vi "All stations screw ID config.vi"(10 "station idx":i32, 11 "configuration file path":path) -> (0 "error out":errorcluster caption="错误输出", 2 "station idx":i32, 3 "configuration file path":path, 5 "Screw config":T1)   [LabVIEW 2018]
uses:
  Crl defs/one state screw config.ctl
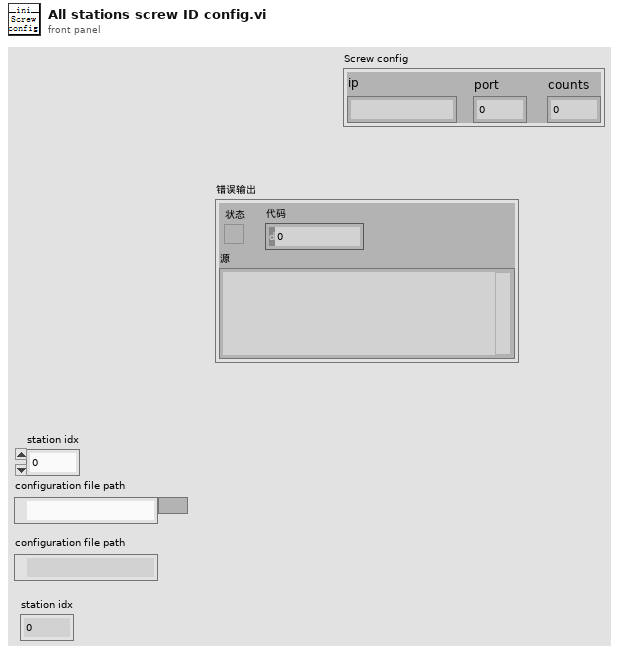
[diagram p1: front panel]
types:
  T1 = typedef "one state screw config.ctl" = cluster{"ip":string, "port":u16, "counts":u16}
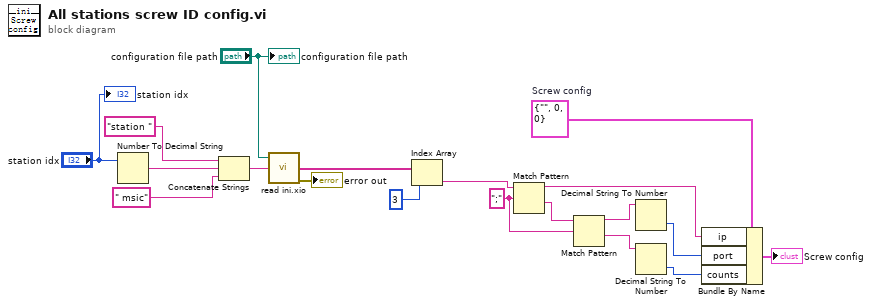
[diagram p0: block diagram]
diagram:
  w7 = T1 {"ip"="", "port"=0, "counts"=0}  # Screw config
  w9 = ";" ("正则表达式")
  n1 = Number To Decimal String(number="station idx") -> (decimal integer string=w17:string)  [unwired: 1 in]
  n2 = Concatenate Strings("station ", w17, " msic" ("string")) -> (w14:string)
  n3 = call "read ini.xio.vi"("configuration file path"="configuration file path", "Sections"=w14) -> ("Values"=w15:string[], "error out"=→"error out":errorcluster)  [unwired: 1 in, 3 out]
  n4 = Index Array(array=w15, index=3 ("索引")) -> (element=w10:string)
  n5 = Match Pattern(string=w10, regular expression=w9) -> (before substring=w6:string, after substring=w8:string)  [unwired: 1 in, 2 out]
  n6 = Match Pattern(string=w8, regular expression=w9) -> (before substring=w5:string, after substring=w4:string)  [unwired: 1 in, 2 out]
  n7 = Decimal String To Number(string=w5) -> (number=w3:i32)  [unwired: 2 in, 1 out]
  n8 = Decimal String To Number(string=w4) -> (number=w2:i32)  [unwired: 2 in, 1 out]
  n9 = Bundle By Name(cluster=w7, "ip"=w6, "port"=w3, "counts"=w2) -> (→"Screw config":T1)
  "configuration file path" <- "configuration file path"
  "station idx" <- "station idx"
